vi "tx + rx.vi"() -> ()   [LabVIEW 2015]
uses:
  <instrlib>/niUSRP/niUSRP Write Tx Data (CDB Cluster).vi
  <vilib>/measure/NI_MABase.lvlib
  <instrlib>/niUSRP/niUSRP Fetch Rx Data (CDB WDT).vi
  <vilib>/measure/NI_MAPro.lvlib
  <vilib>/measure/maspectr.llb/FFT Power Spectrum for 1 Chan (CDB).vi
panel:
  in  "device names 2":refnum<k15>
  out "Baseband Power Spectrum":cluster{"f0":dbl, "df":dbl, "magnitude":dbl[]}(graph)
  in  "stop 2":bool
  in  "active antenna 2":string="RX2"
  out "coerced gain 2":dbl format="%#_6f"
  out "coerced carrier frequency 2":dbl=100000.0 format="%#_6p"
  out "coerced IQ rate 2":dbl=100000.0 format="%#_6p"
  in  "gain 2":dbl=1.0 format="%#_6f"
  in  "carrier frequency 2":dbl=2400000000.0 format="%#_6p"
  in  "IQ rate 2":dbl=1000000.0 format="%#_6p"
  out "coerced gain":dbl=9.999999999999996 format="%#_6f"
  in  "device names":refnum<k15>="192.168.10.2"
  in  "active antenna":string="TX1"
  in  "stop":bool
  in  "timeout":dbl=10.0
  out "coerced carrier frequency":dbl=2000000000.0 format="%#_6p"
  out "coerced IQ rate":dbl=1000000.0 format="%#_6p"
  in  "gain":dbl=10.0 format="%#_6f"
  in  "carrier frequency":dbl=2000000000.0 format="%#_6p"
  in  "IQ rate":dbl=1000000.0 format="%#_6p"
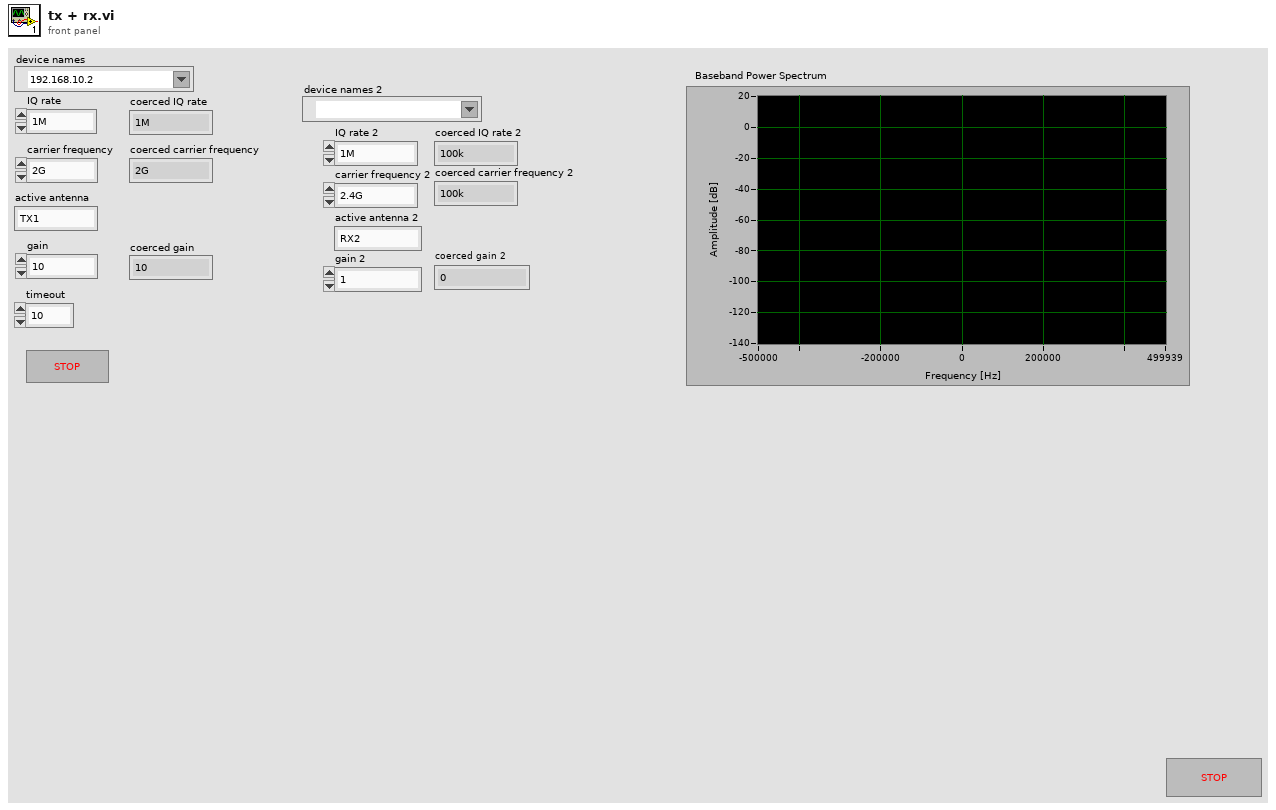
[diagram p1: front panel]
types:
  T1 = typedef "niUSRP Timestamp.ctl" = cluster{"whole seconds":u64, "fractional seconds":dbl}
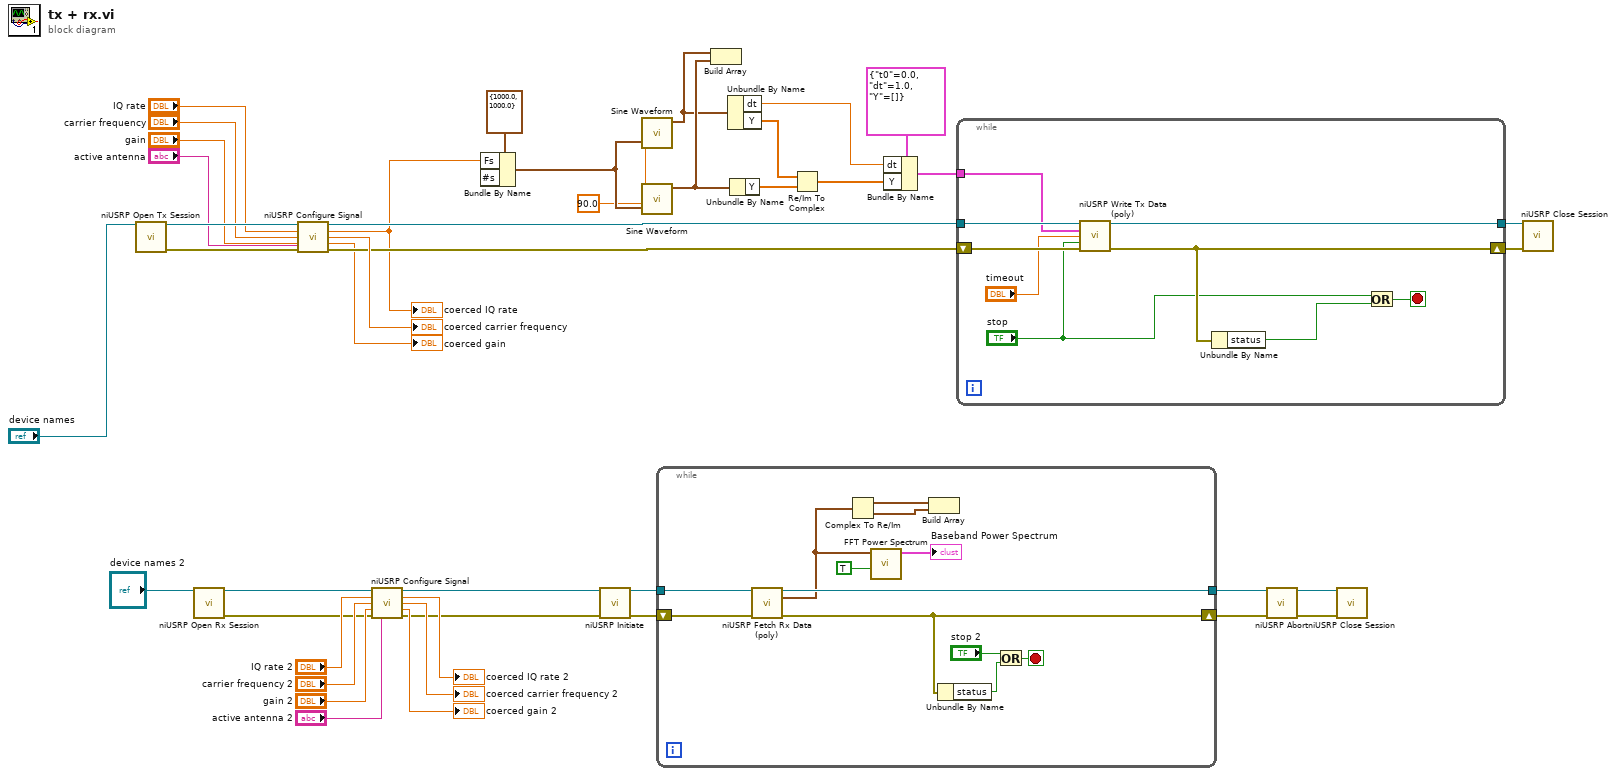
[diagram p0: block diagram]
diagram:
  n1 = call <instrlib>:"niUSRP Open Tx Session.vi"("device names"="device names") -> ("session handle out"=w46:refnum<k15>, "error out"=w43:errorcluster)  [unwired: 13 in]
  n2 = call <instrlib>:"niUSRP Open Rx Session.vi"("device names"="device names 2") -> ("session handle out"=w6:refnum<k15>, "error out"=w5:errorcluster)  [unwired: 13 in]
  n3 = call <instrlib>:"niUSRP Configure Signal.vi"("session handle"=w46, "IQ rate"="IQ rate", "carrier frequency"="carrier frequency", "gain"="gain", "error in (no error)"=w43, "active antenna"="active antenna") -> ("session handle out"=w41:refnum<k15>, "coerced IQ rate"=w35:dbl, "coerced carrier frequency"=→"coerced carrier frequency":dbl, "coerced gain"=→"coerced gain":dbl, "error out"=w40:errorcluster)  [unwired: 5 in]
  "coerced IQ rate" <- w35
  n4 = call <instrlib>:"niUSRP Configure Signal.vi"("session handle"=w6, "IQ rate"="IQ rate 2", "carrier frequency"="carrier frequency 2", "gain"="gain 2", "error in (no error)"=w5, "active antenna"="active antenna 2") -> ("session handle out"=w4:refnum<k15>, "coerced IQ rate"=→"coerced IQ rate 2":dbl, "coerced carrier frequency"=→"coerced carrier frequency 2":dbl, "coerced gain"=→"coerced gain 2":dbl, "error out"=w3:errorcluster)  [unwired: 5 in]
  n5 = Bundle By Name(cluster=cluster{"Fs":dbl, "#s":dbl} {"Fs"=1000.0, "#s"=1000.0} ("sampling info"), "Fs"=w35) -> (w34:cluster{"Fs":dbl, "#s":dbl}, "#s"=w36:dbl)
  n6 = call <instrlib>:"niUSRP Initiate.vi"("session handle"=w4, "error in (no error)"=w3) -> ("session handle out"=w19:refnum<k15>, "error out"=w18:errorcluster)  [unwired: 12 in]
  n7 = call <vilib>:"Sine Waveform.vi"("sampling info"=w34) -> ("signal out"=w30:waveform(dbl), "frequency"=w32:dbl)  [unwired: 8 in, 1 out]
  n8 = call <vilib>:"Sine Waveform.vi"("sampling info"=w34, "phase"=90.0, "frequency"=w32) -> ("signal out"=w31:waveform(dbl))  [unwired: 7 in, 1 out]
  n9 = while {
    tunnel: w19 -> [w62]
    tunnel: [w58] -> w17
    shift-right: [w54] -> w16
    shift-left: w18 -> [w61]
    stop <- w53 stop-if-true
    n10 = call-poly <instrlib>:"niUSRP Fetch Rx Data (poly).vi"("session handle"=w62, "error in (no error)"=w61) -> ("session handle out"=w58:refnum<k15>, "number of samples"=w60:i64, "data"=w51:waveform(cdb), "timeout"=w59:dbl, "timestamp"=w52:T1, "error out"=w54:errorcluster)  [unwired: 8 in]
    n11 = Complex To Re/Im(x + iy=w51) -> (x=w57:waveform(dbl), y=w56:waveform(dbl))
    n12 = call-poly <vilib>:"FFT Power Spectrum.vi"("dB On (F)"=TRUE, "time signal"=w51) -> ("power spectrum"=→"Baseband Power Spectrum":cluster{"f0":dbl, "df":dbl, "magnitude":dbl[]})  [unwired: 6 in, 3 out]
    n13 = Build Array(w57, w56) -> (w55:waveform(dbl)[])
    n14 = Unbundle By Name(w54) -> ("status"=w47:bool)
    n15 = Or(x="stop 2", y=w47) -> (x .or. y?=w53:bool)
  }
  n16 = Build Array(w30, w31) -> (w27:waveform(dbl)[])
  n17 = Unbundle By Name(w30) -> ("dt"=w23:dbl, "Y"=w29:dbl[])
  n18 = Unbundle By Name(w31) -> ("Y"=w28:dbl[])
  n19 = Re/Im To Complex(1:w28, 2:w29) -> (0:w22:cdb[])
  n20 = Bundle By Name(cluster=cluster{"t0":dbl, "dt":dbl, "Y":cdb[]} {"t0"=0.0, "dt"=1.0, "Y"=[]} ("data"), "dt"=w23, "Y"=w22) -> (w21:cluster{"t0":dbl, "dt":dbl, "Y":cdb[]})
  n21 = while {
    tunnel: w41 -> [w70]
    tunnel: [w67] -> w39
    shift-right: [w66] -> w38
    shift-left: w40 -> [w69]
    tunnel: w21 -> [w65]
    stop <- w71 stop-if-true
    n22 = call-poly <instrlib>:"niUSRP Write Tx Data (poly).vi"("session handle"=w70, "data"=w65, "timeout"="timeout", "end of data?"="stop", "error in (no error)"=w69) -> ("session handle out"=w67:refnum<k15>, "error out"=w66:errorcluster)  [unwired: 9 in]
    n23 = Unbundle By Name(w66) -> ("status"=w64:bool)
    n24 = Or(x="stop", y=w64) -> (x .or. y?=w71:bool)
  }
  n25 = call <instrlib>:"niUSRP Abort.vi"("session handle"=w17, "error in (no error)"=w16) -> ("session handle out"=w14:refnum<k15>, "error out"=w15:errorcluster)  [unwired: 12 in]
  n26 = call <instrlib>:"niUSRP Close Session.vi"("session handle"=w14, "error in (no error)"=w15) -> ()  [unwired: 13 in, 1 out]
  n27 = call <instrlib>:"niUSRP Close Session.vi"("session handle"=w39, "error in (no error)"=w38) -> ()  [unwired: 13 in, 1 out]
